vi "trash_CIF Manager U_BUI.vi"() -> ()   [LabVIEW 2021]
uses:
  CIFUI/Typedef/New Plugin.ctl
  CIFUI/Typedef/Channel Connection.ctl
  CIFUI/CIF_UI.lvclass
  CIFPluginManager/gRPC/CIF_Manager_Client_Wrapper/CIFManagerClientWrapper.lvlib
  CIFUI/Typedef/Direction to Include.ctl
  CIFUI/Typedef/Core UI References.ctl
  CIFPluginManager/gRPC/CIF_Manager_client/RPC Messages/cif_manager_OrchestrationLanguage.ctl
  CIFPluginManager/gRPC/CIF_Manager_client/CIF_Manager_client.lvlib
  CIFPluginManager/gRPC/CIF_Manager_client/RPC Messages/cif_manager_OrchConfig.ctl
panel:
  in  "Tab Control":T1(tab)
  in  "Link Channel":bool
  in  "Connection":T2
  in  "Subscriber Channels":string(tree)
  in  "Publisher Channels":string(tree)
  in  "New Plugin":T3={"Unique Name"="test", "Type"="", "Version (Optional)"=""}
  in  "Loaded Plugins":string(tree)
  in  "Update Plugin Types":bool
  in  "EXIT":bool
  in  "Discovered Plugins":string(tree)
  in  "Load Plugin":bool
  in  "Abort Plugin":bool
  in  "Plugin to abort":string
  in  "Abort All Plugins":bool
  in  "address":string="192.168.1.160"
  in  "Reset Info":bool
  out "Info":string
  out "Errors Present":bool
  in  "Get All Info":bool
  out "Plugin Address":string
  out "Connected":bool
  in  "Connection 2":bool
  in  "Plugin Status":string[][](table)
  out "Orchestration":string
  in  "Generate Orchestration":bool
  in  "Errors 2":i32(listbox)=-1
  in  "Reset Errors":bool
  in  "Clear Local":bool
  out "Config":string
  in  "Get Config":bool
  in  "Reset Config":bool
  in  "Get All Errors":bool
  in  "All Config":bool
  out "Error Message":string
  in  "File Name":string="orchestrate.py"
  in  "Start Timestamp":u64
  in  "Session Id":u64
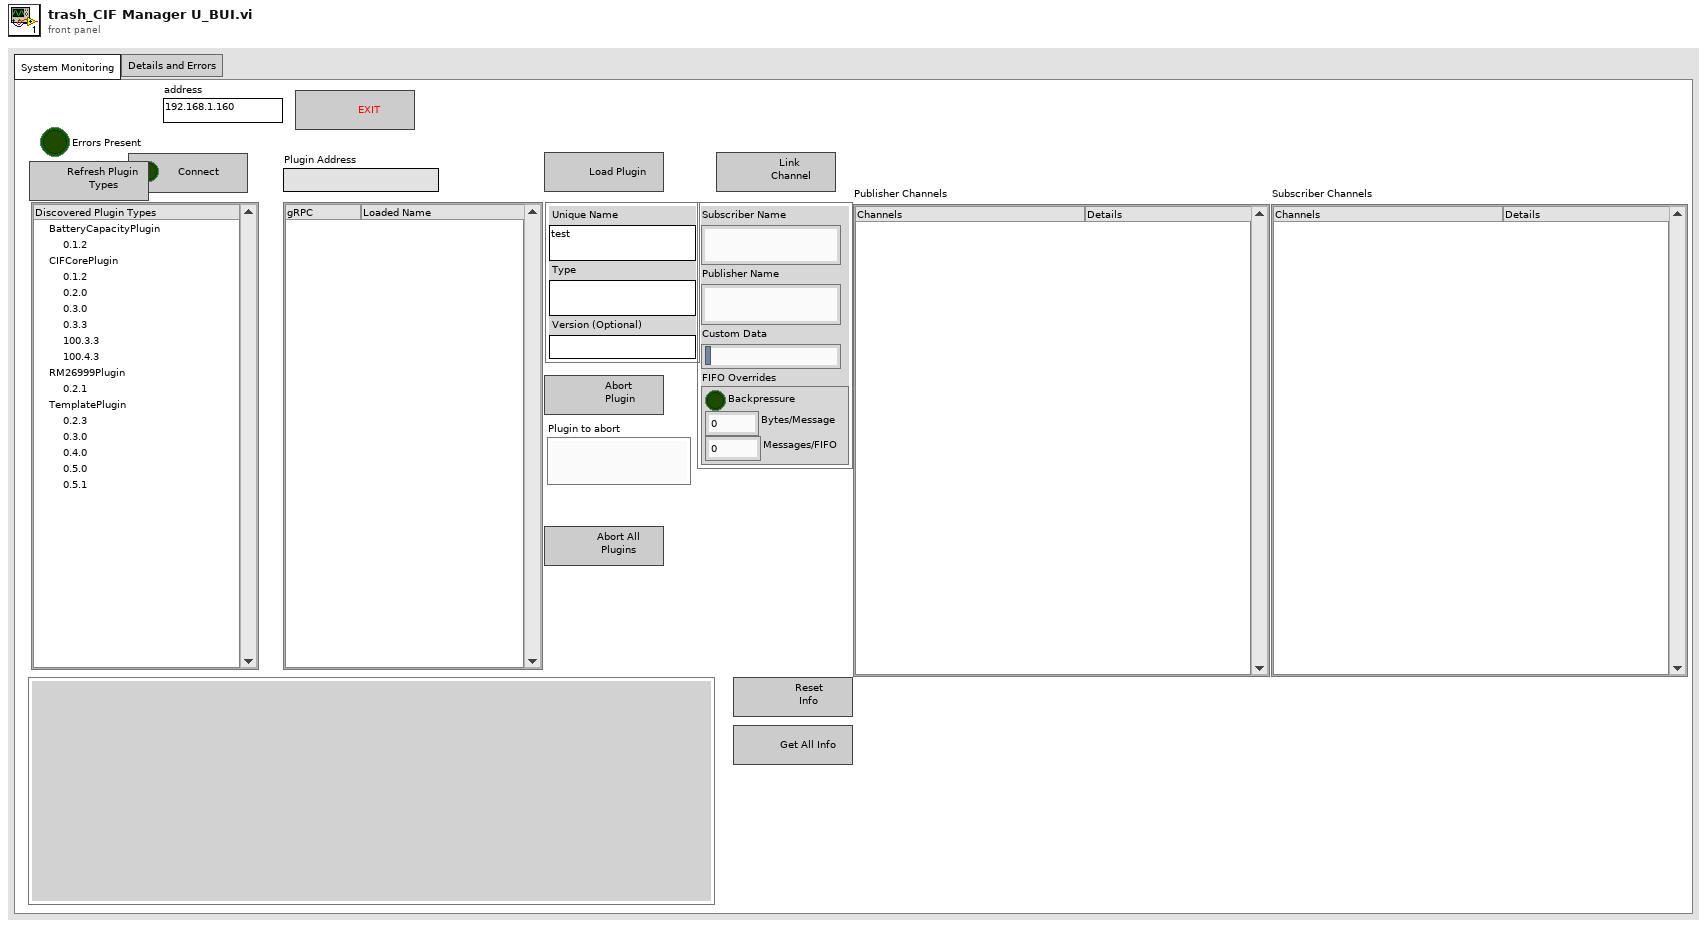
[diagram p1: front panel]
types:
  T1 = enum32{"System Monitoring", "Details and Errors"}
  T2 = typedef "CIF_UI.lvclass/Channel Connection.ctl" = cluster{"Subscriber Name":string, "Publisher Name":string, "Custom Data":string, "FIFO Overrides":cluster{"Backpressure":bool, "Bytes/Message":u32, "Messages/FIFO":u32}}
  T3 = typedef "CIF_UI.lvclass/New Plugin.ctl" = cluster{"Unique Name":string, "Type":string, "Version (Optional)":string}
  T4 = typedef "CIF_UI.lvclass/Core UI References.ctl" = cluster{"Discovered Plugins":refnum<vi>, "Discovered Plugins Valid":bool, "Loaded Plugins":refnum<vi>, "Loaded Plugins Valid":bool, "Publisher Channels":refnum<vi>, "Publisher Channels Valid":bool, "Subscriber Channels":refnum<vi>, "Subscriber Channels Valid":bool, "Plugin Status":refnum<vi>, "Plugin Status Valid":bool, "Channel Connection":refnum<vi>, "Channel Connection Valid":bool, "New Plugin Load":refnum<vi>, "New Plugin Load Valid":bool, "Errors":refnum<vi>, "Errors Valid":bool, "Plugin to Abort":refnum<vi>, "Plugin to Abort Valid":bool, "Connection":refnum<vi>, "Connection Valid":bool, "Exit":refnum<vi>, "Exit Valid":bool, "Run Listen":refnum<vi>, "Run Listen Valid":bool, "CIF Manager Tab":refnum<vi>, "Manger Tab Valid":bool, "Clear Local Error":refnum<vi>, "Clear Local Error Valid":bool, "Local Error":refnum<vi>, "Local Error Valid":bool, "System Errors":refnum<vi>, "System Errors Valid":bool, "Plugin Selection":refnum<vi>, "Plugin Selection Valid":bool}
  T5 = typedef "CIF_UI.lvclass/Direction to Include.ctl" = enum16{"All", "Subscriber", "Publisher"}
  T6 = typedef "CIF_Manager_client.lvlib/cif_manager_OrchConfig.ctl" = cluster{"start_timestamp":u64, "create_file":bool, "orchestration_language":T7, "filename":string, "default_ip":string}
  T7 = typedef "CIF_Manager_client.lvlib/cif_manager_OrchestrationLanguage.ctl" = enum32{"NULL", "PYTHON"}
  T8 = typedef "InstrumentStudio Plugin SDK.lvlib/Event Registration Refnum.ctl" = refnum<event-registration>
  T9 = typedef "grpc-lvsupport-release.lvlib/grpcId.ctl" = u64
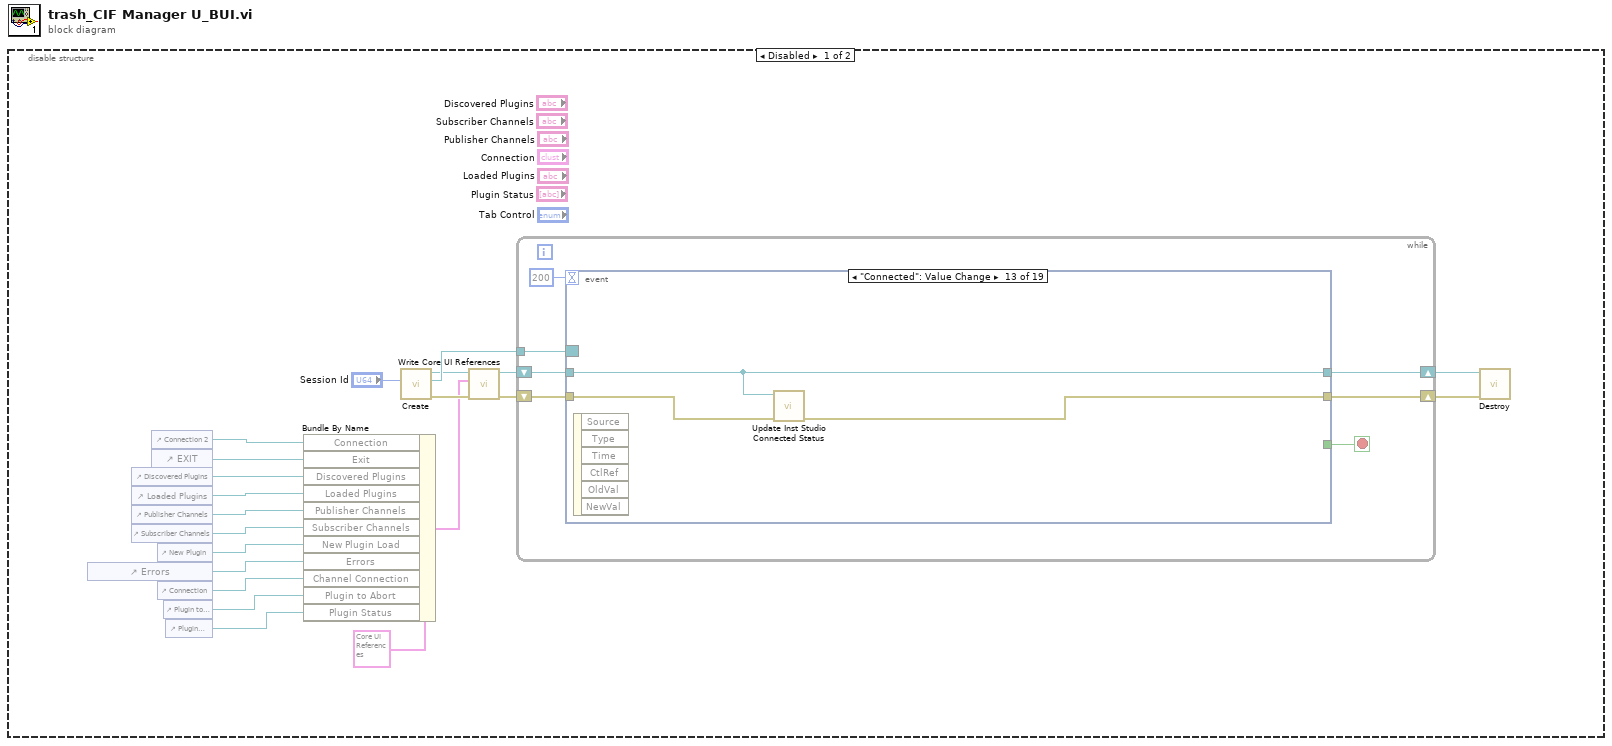
[diagram p0: block diagram]
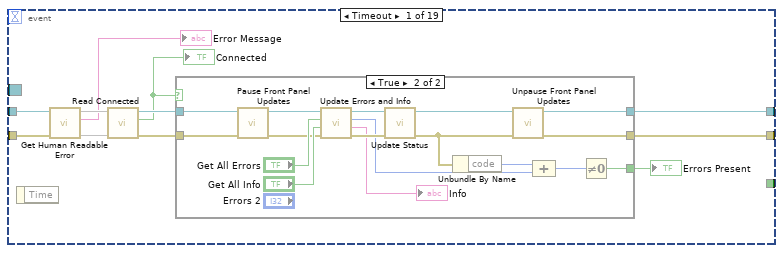
[diagram p2: hidden frame]
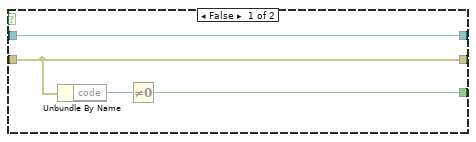
[diagram p3: hidden frame]
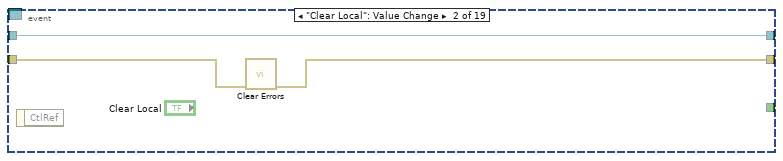
[diagram p4: hidden frame]
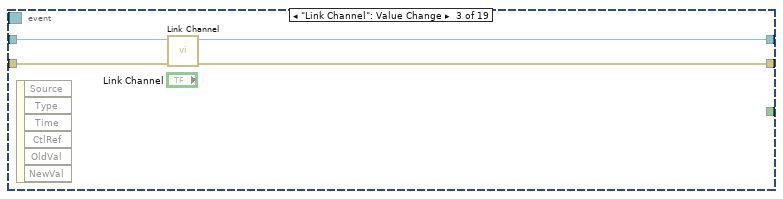
[diagram p5: hidden frame]
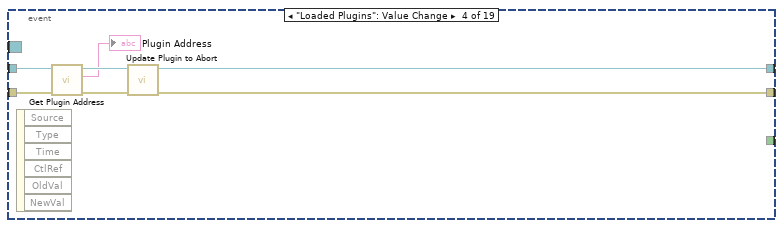
[diagram p6: hidden frame]
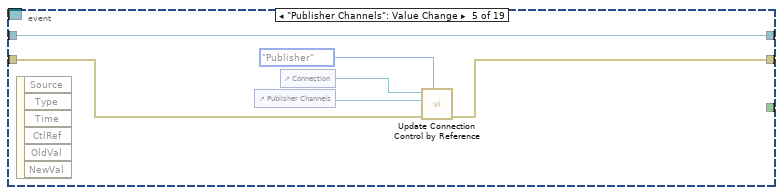
[diagram p7: hidden frame]
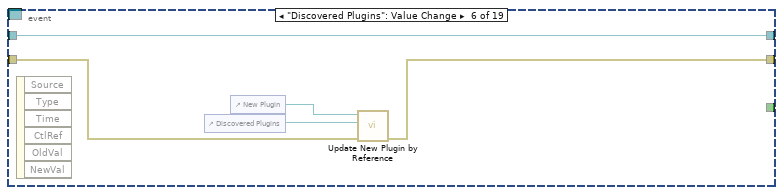
[diagram p8: hidden frame]
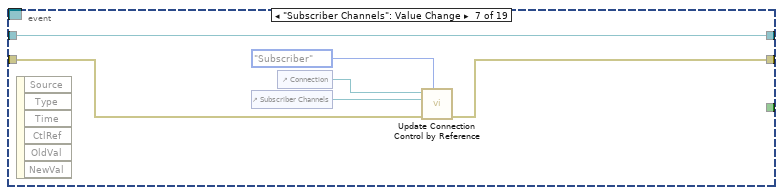
[diagram p9: hidden frame]
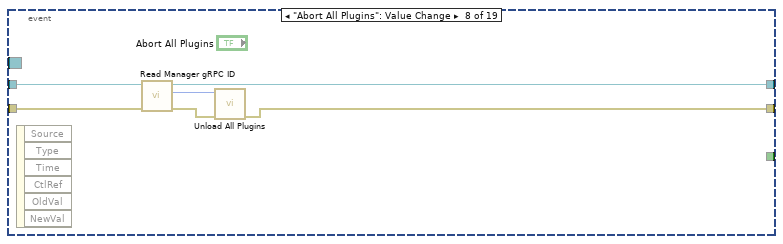
[diagram p10: hidden frame]
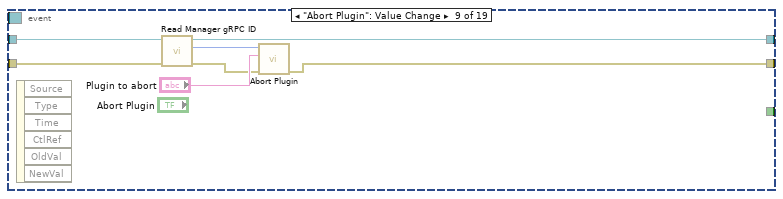
[diagram p11: hidden frame]
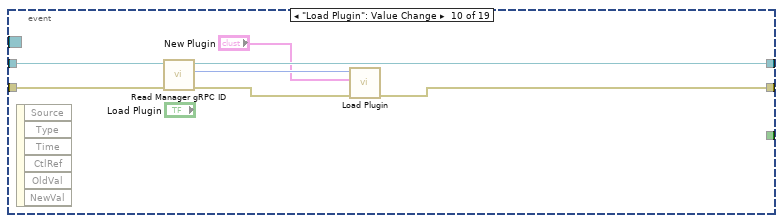
[diagram p12: hidden frame]
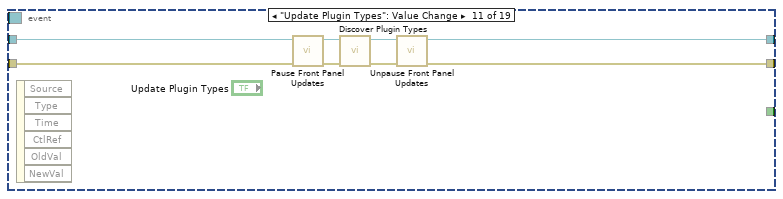
[diagram p13: hidden frame]
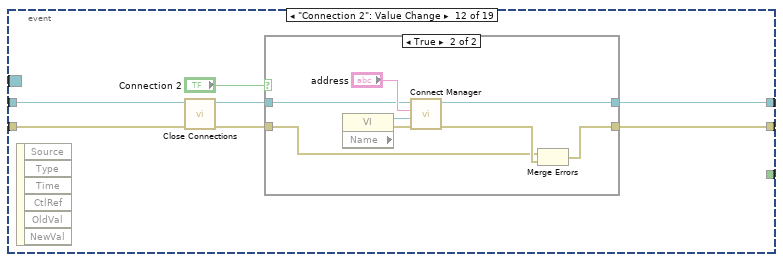
[diagram p14: hidden frame]
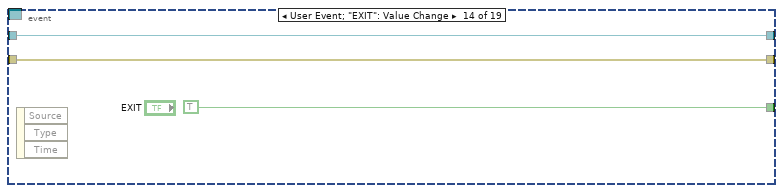
[diagram p16: hidden frame]
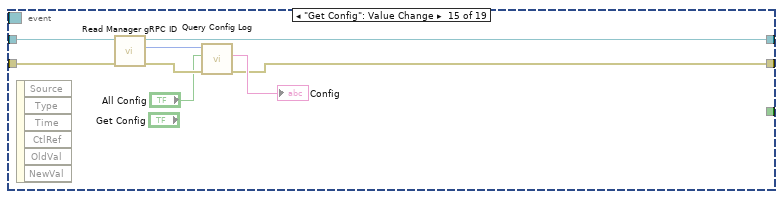
[diagram p17: hidden frame]
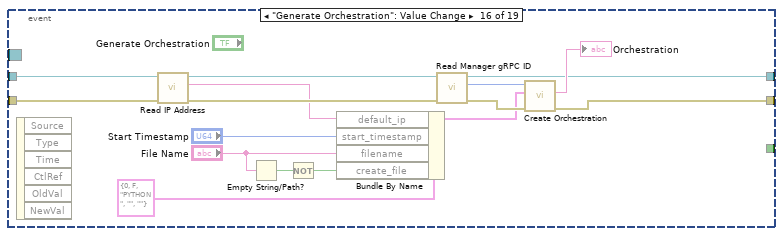
[diagram p18: hidden frame]
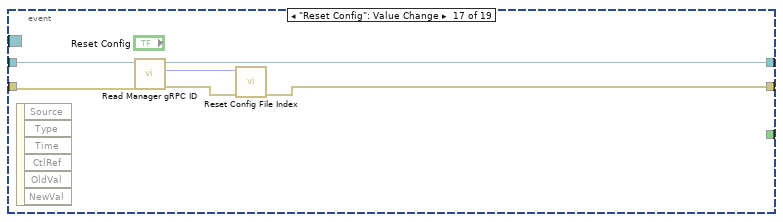
[diagram p19: hidden frame]
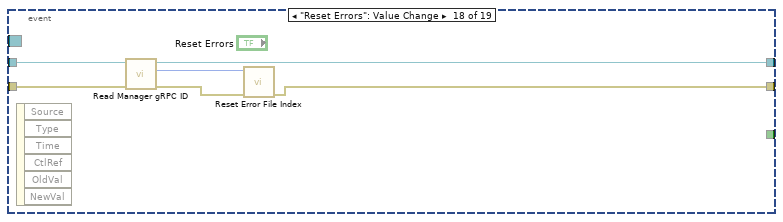
[diagram p20: hidden frame]
diagram:
  n1 = disable-structure shown="Disabled" {
    frame Disabled {
      n2 = control-ref of="Errors"() -> (w14:refnum<vi>)
      n3 = control-ref of="Discovered Plugins"() -> (w19:refnum<vi>)
      n4 = control-ref of="Loaded Plugins"() -> (w18:refnum<vi>)
      n5 = control-ref of="Publisher Channels"() -> (w17:refnum<vi>)
      n6 = control-ref of="Subscriber Channels"() -> (w16:refnum<vi>)
      n7 = control-ref of="Connection 2"() -> (w2:refnum<vi>)
      n8 = control-ref of="EXIT"() -> (w3:refnum<vi>)
      n9 = control-ref of="New Plugin"() -> (w15:refnum<vi>)
      n10 = control-ref of="Connection"() -> (w13:refnum<vi>)
      n11 = control-ref of="Plugin to abort"() -> (w12:refnum<vi>)
      n12 = control-ref of="Plugin Status"() -> (w1:refnum<vi>)
      n13 = Bundle By Name(cluster=T4 {"Discovered Plugins"=refnum, "Discovered Plugins Valid"=FALSE, "Loaded Plugins"=refnum, "Loaded Plugins Valid"=FALSE, "Publisher Channels"=refnum, "Publisher Channels Valid"=FALSE, "Subscriber Channels"=refnum, "Subscriber Channels Valid"=FALSE, "Plugin Status"=refnum, "Plugin Status Valid"=FALSE, "Channel Connection"=refnum, "Channel Connection Valid"=FALSE, "New Plugin Load"=refnum, "New Plugin Load Valid"=FALSE, "Errors"=refnum, "Errors Valid"=FALSE, "Plugin to Abort"=refnum, "Plugin to Abort Valid"=FALSE, "Connection"=refnum, "Connection Valid"=FALSE, "Exit"=refnum, "Exit Valid"=FALSE, "Run Listen"=refnum, "Run Listen Valid"=FALSE, "CIF Manager Tab"=refnum, "Manger Tab Valid"=FALSE, "Clear Local Error"=refnum, "Clear Local Error Valid"=FALSE, "Local Error"=refnum, "Local Error Valid"=FALSE, "System Errors"=refnum, "System Errors Valid"=FALSE, "Plugin Selection"=refnum, "Plugin Selection Valid"=FALSE} ("UI References"), "Connection"=w2, "Exit"=w3, "Discovered Plugins"=w19, "Loaded Plugins"=w18, "Publisher Channels"=w17, "Subscriber Channels"=w16, "New Plugin Load"=w15, "Errors"=w14, "Channel Connection"=w13, "Plugin to Abort"=w12, "Plugin Status"=w1) -> (w4:T4)
      n14 = call "Create.vi"("Session Id"="Session Id") -> ("error out"=w7:errorcluster, "Event Refnum"=w11:T8, "CIF_UI out"=w8:refnum<class "CIF_UI.lvclass">)  [unwired: 8 in]
      n15 = call "Write Core UI References.vi"("error in (no error)"=w7, "UI References"=w4, "CIF_UI in"=w8) -> ("error out"=w5:errorcluster, "CIF_UI out"=w6:refnum<class "CIF_UI.lvclass">)  [unwired: 7 in]
      n16 = while {
        tunnel: w11 -> [w27]
        shift-right: [w22] -> w20
        shift-left: w6 -> [w25]
        shift-right: [w23] -> w21
        shift-left: w5 -> [w24]
        stop <- w26 stop-if-true
        n17 = event shown="[12] \"Connected\": Value Change" {
          selector: w27 -> [_ _ _ _ _ _ _ _ _ _ _ _ _ _ _ _ _ _ _]
          dyn-events: _ -> [_ _ _ _ _ _ _ _ _ _ _ _ _ _ _ _ _ _ _]
          timeout: 200 -> [_ _ _ _ _ _ _ _ _ _ _ _ _ _ _ _ _ _ _]
          tunnel: [_ _ _ _ _ _ _ _ _ _ _ _ _ TRUE _ _ _ _ _] -> w26
          tunnel: w25 -> [w34 w61 w67 w72 w75 w81 w87 w95 w102 w109 w119 w124 w137 w141 w146 w161 w170 w176 w182]
          tunnel: w24 -> [w33 w63 w66 w71 w77 w85 w89 w94 w101 w108 w118 w123 w139 w140 w145 w160 w169 w175 w181]
          tunnel: [w35 w62 w65 w74 w76 w82 w88 w93 w98 w107 w112 w125 w138 w140 w144 w165 w167 w173 w179] -> w23
          tunnel: [w39 w61 w64 w73 w75 w81 w87 w92 w99 w106 w113 w126 w137 w141 w143 w163 w168 w174 w180] -> w22
          event Timeout {
            n18 = event-data() -> ()  [unwired: 1 in, 1 out]
            n19 = call "Get Human Readable Error.vi"("error in (no error)"=w33, 11:w34) -> (0:w32, "Error Message"=→"Error Message":string, 3:w31)  [unwired: 7 in]
            n20 = call "Read Connected.vi"("error in (no error)"=w32, "CIF_UI in"=w31) -> ("error out"=w36:errorcluster, "Connected"=w29:bool, "CIF_UI out"=w37:refnum<class "CIF_UI.lvclass">)  [unwired: 7 in]
            "Connected" <- w29
            n21 = case shown="True" w29 {
              tunnel: w36 -> [w42 w46]
              tunnel: [w42 w49] -> w35
              tunnel: w37 -> [w43 w47]
              tunnel: [w43 w48] -> w39
              tunnel: [w40 w58] -> w38
              frame False {
                n22 = Unbundle By Name(w42) -> ("code"=w41:i32)
                n23 = Not Equal To 0?(x=w41) -> (x != 0?=w40:bool)
              }
              frame True {
                n24 = call "Pause Front Panel Updates.vi"("error in (no error)"=w46, "CIF_UI in"=w47) -> ("error out"=w44:errorcluster, "CIF_UI out"=w45:refnum<class "CIF_UI.lvclass">)  [unwired: 8 in]
                n25 = call "Update Errors and Info.vi"("error in (no error)"=w44, "Get All Info"="Get All Info", "Get All Errors"="Get All Errors", "CIF_UI in"=w45) -> ("error out"=w57:errorcluster, "Info"=→"Info":string, "Error Count"=w53:i32, "CIF_UI out"=w56:refnum<class "CIF_UI.lvclass">)  [unwired: 4 in]
                n26 = call "Update Status.vi"("error in (no error)"=w57, "CIF_UI in"=w56) -> ("error out"=w50:errorcluster, "CIF_UI out"=w51:refnum<class "CIF_UI.lvclass">)  [unwired: 8 in]
                n27 = Unbundle By Name(w50) -> ("code"=w60:i32)
                n28 = call "Unpause Front Panel Updates.vi"("error in (no error)"=w50, "CIF_UI in"=w51) -> ("error out"=w49:errorcluster, "CIF_UI out"=w48:refnum<class "CIF_UI.lvclass">)  [unwired: 8 in]
                n29 = Compound Arithmetic op=ADD(w60, w53) -> (w59:i32)
                n30 = Not Equal To 0?(x=w59) -> (x != 0?=w58:bool)
              }
            }
            "Errors Present" <- w38
          }
          event "Clear Local": Value Change {
            n31 = event-data() -> ()  [unwired: 1 in, 1 out]
            n32 = call <vilib>:"Clear Errors.vi"("error in (no error)"=w63) -> ("error out"=w62:errorcluster)  [unwired: 5 in, 1 out]
          }
          event "Link Channel": Value Change {
            n33 = event-data() -> ()  [unwired: 1 in, 6 out]
            n34 = call "Link Channel.vi"("error in (no error)"=w66, "CIF_UI in"=w67) -> ("error out"=w65:errorcluster, "CIF_UI out"=w64:refnum<class "CIF_UI.lvclass">)  [unwired: 8 in]
          }
          event "Loaded Plugins": Value Change {
            n35 = event-data() -> ()  [unwired: 1 in, 6 out]
            n36 = call "Get Plugin Address.vi"("error in (no error)"=w71, "CIF_UI in"=w72) -> ("error out"=w69:errorcluster, "Plugin Address"=→"Plugin Address":string, "CIF_UI out"=w70:refnum<class "CIF_UI.lvclass">)  [unwired: 7 in]
            n37 = call "Update Plugin to Abort.vi"("error in (no error)"=w69, "CIF_UI in"=w70) -> ("error out"=w74:errorcluster, "CIF_UI out"=w73:refnum<class "CIF_UI.lvclass">)  [unwired: 8 in]
          }
          event "Publisher Channels": Value Change {
            n38 = event-data() -> ()  [unwired: 1 in, 6 out]
            n39 = control-ref of="Publisher Channels"() -> (w78:refnum<vi>)
            n40 = control-ref of="Connection"() -> (w79:refnum<vi>)
            n41 = call "Update Connection Control by Reference.vi"("Direction to Include"=Direction_to_Include."Publisher", "error in (no error)"=w77, "Channels"=w78, "Channel Connection"=w79) -> ("error out"=w76:errorcluster)  [unwired: 6 in, 1 out]
          }
          event "Discovered Plugins": Value Change {
            n42 = event-data() -> ()  [unwired: 1 in, 6 out]
            n43 = control-ref of="Discovered Plugins"() -> (w83:refnum<vi>)
            n44 = control-ref of="New Plugin"() -> (w84:refnum<vi>)
            n45 = call "Update New Plugin by Reference.vi"("error in (no error)"=w85, "Plugin Types Tree"=w83, "New Plugin Control"=w84) -> ("error out"=w82:errorcluster)  [unwired: 8 in]
          }
          event "Subscriber Channels": Value Change {
            n46 = event-data() -> ()  [unwired: 1 in, 6 out]
            n47 = control-ref of="Subscriber Channels"() -> (w86:refnum<vi>)
            n48 = control-ref of="Connection"() -> (w90:refnum<vi>)
            n49 = call "Update Connection Control by Reference.vi"("Direction to Include"=Direction_to_Include."Subscriber", "error in (no error)"=w89, "Channels"=w86, "Channel Connection"=w90) -> ("error out"=w88:errorcluster)  [unwired: 6 in, 1 out]
          }
          event "Abort All Plugins": Value Change {
            n50 = event-data() -> ()  [unwired: 1 in, 6 out]
            n51 = call "Read Manager gRPC ID.vi"("error in (no error)"=w94, "CIF_UI in"=w95) -> ("error out"=w96:errorcluster, "Manager gRPCid"=w97:T9, "CIF_UI out"=w92:refnum<class "CIF_UI.lvclass">)  [unwired: 7 in]
            n52 = call "Unload All Plugins.vi"("error in"=w96, "gRPC ID in"=w97) -> ("error out"=w93:errorcluster)  [unwired: 8 in, 1 out]
          }
          event "Abort Plugin": Value Change {
            n53 = event-data() -> ()  [unwired: 1 in, 6 out]
            n54 = call "Read Manager gRPC ID.vi"("error in (no error)"=w101, "CIF_UI in"=w102) -> ("error out"=w100:errorcluster, "Manager gRPCid"=w104:T9, "CIF_UI out"=w99:refnum<class "CIF_UI.lvclass">)  [unwired: 7 in]
            n55 = call "Abort Plugin.vi"("error in"=w100, "plugin_name"="Plugin to abort", "gRPC ID in"=w104) -> ("error out"=w98:errorcluster)  [unwired: 7 in, 1 out]
          }
          event "Load Plugin": Value Change {
            n56 = event-data() -> ()  [unwired: 1 in, 6 out]
            n57 = call "Read Manager gRPC ID.vi"("error in (no error)"=w108, "CIF_UI in"=w109) -> ("error out"=w110:errorcluster, "Manager gRPCid"=w111:T9, "CIF_UI out"=w106:refnum<class "CIF_UI.lvclass">)  [unwired: 7 in]
            n58 = call "Load Plugin.vi"("error in"=w110, "New Plugin"="New Plugin", "gRPC ID in"=w111) -> ("error out"=w107:errorcluster)  [unwired: 7 in, 1 out]
          }
          event "Update Plugin Types": Value Change {
            n59 = event-data() -> ()  [unwired: 1 in, 6 out]
            n60 = call "Pause Front Panel Updates.vi"("error in (no error)"=w118, "CIF_UI in"=w119) -> ("error out"=w117:errorcluster, "CIF_UI out"=w116:refnum<class "CIF_UI.lvclass">)  [unwired: 8 in]
            n61 = call "Discover Plugin Types.vi"("error in (no error)"=w117, "CIF_UI in"=w116) -> ("error out"=w114:errorcluster, "CIF_UI out"=w115:refnum<class "CIF_UI.lvclass">)  [unwired: 8 in]
            n62 = call "Unpause Front Panel Updates.vi"("error in (no error)"=w114, "CIF_UI in"=w115) -> ("error out"=w112:errorcluster, "CIF_UI out"=w113:refnum<class "CIF_UI.lvclass">)  [unwired: 8 in]
          }
          event "Connection 2": Value Change {
            n63 = event-data() -> ()  [unwired: 1 in, 6 out]
            n64 = call "Close Connections.vi"("error in (no error)"=w123, "CIF_UI in"=w124) -> ("error out"=w122:errorcluster, "CIF_UI out"=w121:refnum<class "CIF_UI.lvclass">)  [unwired: 8 in]
            n65 = case shown="True" "Connection 2" {
              tunnel: [w128 w132] -> w126
              tunnel: [w127 w131] -> w125
              tunnel: w122 -> [w127 w130]
              tunnel: w121 -> [w128 w129]
              frame False {
              }
              frame True {
                n66 = property class="VI" props=["Name"]() -> (reference out=w136:refnum<vi>, error out=w135:errorcluster)  [unwired: 2 in, 1 out]
                n67 = call "Connect Manager.vi"("error in (no error)"=w135, "VI Reference"=w136, "Address"="address", "CIF_UI in"=w129) -> ("error out"=w133:errorcluster, "CIF_UI out"=w132:refnum<class "CIF_UI.lvclass">)  [unwired: 6 in]
                n68 = Merge Errors(w130, w133) -> (w131:errorcluster)
              }
            }
          }
          event "Connected": Value Change {
            n69 = event-data() -> ()  [unwired: 1 in, 6 out]
            n70 = call "Update Inst Studio Connected Status.vi"("error in (no error)"=w139, "CIF_UI in"=w137) -> ("error out"=w138:errorcluster)  [unwired: 9 in]
          }
          event User Event; "EXIT": Value Change {
            n71 = event-data() -> ()  [unwired: 1 in, 3 out]
          }
          event "Get Config": Value Change {
            n72 = event-data() -> ()  [unwired: 1 in, 6 out]
            n73 = call "Read Manager gRPC ID.vi"("error in (no error)"=w145, "CIF_UI in"=w146) -> ("error out"=w149:errorcluster, "Manager gRPCid"=w150:T9, "CIF_UI out"=w143:refnum<class "CIF_UI.lvclass">)  [unwired: 7 in]
            n74 = call "Query Config Log.vi"("error in"=w149, "query_all"="All Config", "gRPC ID in"=w150) -> ("error out"=w144:errorcluster, "Config"=→"Config":string)  [unwired: 6 in, 1 out]
          }
          event "Generate Orchestration": Value Change {
            n75 = event-data() -> ()  [unwired: 1 in, 6 out]
            n76 = call "Read IP Address.vi"("error in (no error)"=w160, "CIF_UI in"=w161) -> ("error out"=w158:errorcluster, "IP address"=w155:string, "CIF_UI out"=w159:refnum<class "CIF_UI.lvclass">)  [unwired: 7 in]
            n77 = Empty String/Path?(string/path="File Name") -> (empty?=w153:bool)
            n78 = Not(x=w153) -> (.not. x?=w152:bool)
            n79 = Bundle By Name(cluster=T6 {"start_timestamp"=0, "create_file"=FALSE, "orchestration_language"=enum."PYTHON", "filename"="", "default_ip"=""} ("Orchestration Config"), "default_ip"=w155, "start_timestamp"="Start Timestamp", "filename"="File Name", "create_file"=w152) -> (w156:T6)
            n80 = call "Read Manager gRPC ID.vi"("error in (no error)"=w158, "CIF_UI in"=w159) -> ("error out"=w162:errorcluster, "Manager gRPCid"=w166:T9, "CIF_UI out"=w163:refnum<class "CIF_UI.lvclass">)  [unwired: 7 in]
            n81 = call "Create Orchestration.vi"("error in"=w162, "Orchestration Config"=w156, "gRPC ID in"=w166) -> ("error out"=w165:errorcluster, "Orchestration Script"=→"Orchestration":string)  [unwired: 6 in, 1 out]
          }
          event "Reset Config": Value Change {
            n82 = event-data() -> ()  [unwired: 1 in, 6 out]
            n83 = call "Read Manager gRPC ID.vi"("error in (no error)"=w169, "CIF_UI in"=w170) -> ("error out"=w171:errorcluster, "Manager gRPCid"=w172:T9, "CIF_UI out"=w168:refnum<class "CIF_UI.lvclass">)  [unwired: 7 in]
            n84 = call "Reset Config File Index.vi"("error in"=w171, "gRPC ID in"=w172) -> ("error out"=w167:errorcluster)  [unwired: 8 in, 1 out]
          }
          event "Reset Errors": Value Change {
            n85 = event-data() -> ()  [unwired: 1 in, 6 out]
            n86 = call "Read Manager gRPC ID.vi"("error in (no error)"=w175, "CIF_UI in"=w176) -> ("error out"=w177:errorcluster, "Manager gRPCid"=w178:T9, "CIF_UI out"=w174:refnum<class "CIF_UI.lvclass">)  [unwired: 7 in]
            n87 = call "Reset Error File Index.vi"("error in"=w177, "gRPC ID in"=w178) -> ("error out"=w173:errorcluster)  [unwired: 8 in, 1 out]
          }
          event "Reset Info": Value Change {
            n88 = event-data() -> ()  [unwired: 1 in, 6 out]
            n89 = call "Read Manager gRPC ID.vi"("error in (no error)"=w181, "CIF_UI in"=w182) -> ("error out"=w183:errorcluster, "Manager gRPCid"=w184:T9, "CIF_UI out"=w180:refnum<class "CIF_UI.lvclass">)  [unwired: 7 in]
            n90 = call "Reset Info File Index.vi"("error in"=w183, "gRPC ID in"=w184) -> ("error out"=w179:errorcluster)  [unwired: 8 in, 1 out]
          }
        }
      }
      n91 = call "Destroy.vi"("error in (no error)"=w21, "CIF_UI in"=w20) -> ()  [unwired: 8 in, 2 out]
    }
    frame Enabled {
    }
  }
